vi "toNextWeekDay.vi"(11 "Cron in":T1) -> (3 "Cron out":T1)   [LabVIEW 2013, in "openCron.lvlib" / "Cron.lvclass"]
uses:
  Cron.lvclass
  CronTime -- cluster.ctl
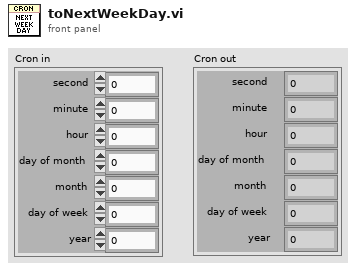
[diagram p1: front panel]
types:
  T1 = typedef "openCron.lvlib/Cron.lvclass/CronTime -- cluster.ctl" = cluster{"second":i32, "minute":i32, "hour":i32, "day of month":i32, "month":i32, "day of week":i32, "year":i32}
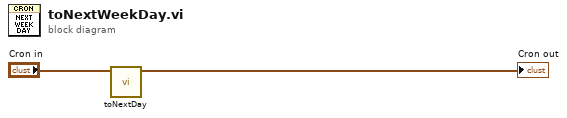
[diagram p0: block diagram]
diagram:
  n1 = call "toNextDay.vi"("Cron in"="Cron in") -> ("Cron out"=→"Cron out":T1)  [unwired: 10 in]
